vi "CurrentOutput_flt.vi"(7 "y scaled":dbl, 9 "array":dbl[][](array[numeric]), 10 "Z Input":dbl, 11 "X Input":dbl) -> (3 "Current Out":dbl)   [LabVIEW 2017]
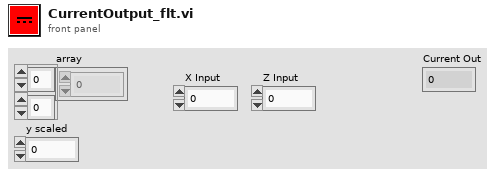
[diagram p1: front panel]
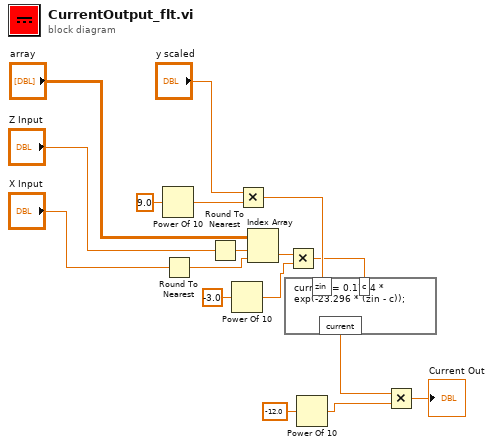
[diagram p0: block diagram]
diagram:
  n1 = Power Of 10(x=9.0) -> (10^x=w13:dbl)
  n2 = Round To Nearest(number="X Input") -> (nearest integer value=w7:dbl)
  n3 = Round To Nearest(number="Z Input") -> (nearest integer value=w15:dbl)
  n4 = Power Of 10(x=-3.0) -> (10^x=w9:dbl)
  n5 = Multiply(x="y scaled", y=w13) -> (x*y=w11:dbl)
  n6 = Index Array(array="array", index (row)=w15, index (col)=w7) -> (element=w4:dbl)
  n7 = Multiply(x=w4, y=w9) -> (x*y=w8:dbl)
  n8 = formula code="current = 0.1714 * exp(-23.296 * (zin - c));"("zin"=w11, "c"=w8) -> ("current"=w14:dbl)
  n9 = Power Of 10(x=-12.0) -> (10^x=w17:dbl)
  n10 = Multiply(x=w14, y=w17) -> (x*y=→"Current Out":dbl)
